vi "Create Master Instance (UDP).vi"(4 "write operation timeout":i32=1000, 6 "read operation timeout":i32=1000, 8 "error in (no error)":errorcluster, 9 "connect timeout":i32=1000, 10 "port (auto)":u16, 11 "address":string) -> (0 "error out":errorcluster, 3 "UDP master instance":refnum<class "Modbus Master.lvclass">)   [LabVIEW 2021]
doc: "Creates a serial or TCP Modbus master instance. You must manually select the polymorphic instance to use."
uses:
  Modbus Master.lvclass
  Modbus_v2/subvis/Transmission Data Unit (ADU)/IP Data Unit/IP Data Unit.lvclass
  Modbus API.lvclass
  Transmission Data Unit/Transmission Data Unit.lvclass
  Modbus_v2/subvis/Protocol/UDP/UDP Master/UDP Master.lvclass
  D:/my_projects/projects/Algorithms/Labview/21/Modbus_v21/API/Modbus API.lvclass
  D:/my_projects/projects/Algorithms/Labview/21/Modbus_v21/API/Master/Modbus Master.lvclass
  Network Protocol/Network Master/Network Master.lvclass
  D:/my_projects/projects/Algorithms/Labview/21/Modbus_v21/Network Protocol/Network Protocol.lvclass
  D:/my_projects/projects/Algorithms/Labview/21/Modbus_v21/Network Protocol/Network Master/Network Master.lvclass
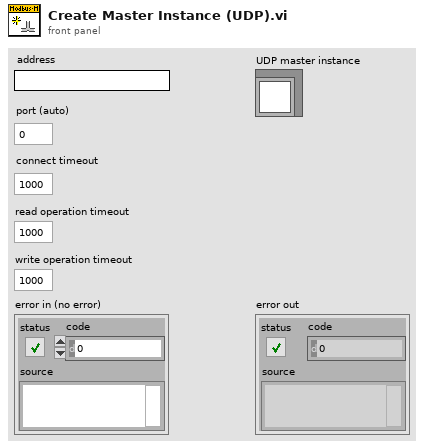
[diagram p1: front panel]
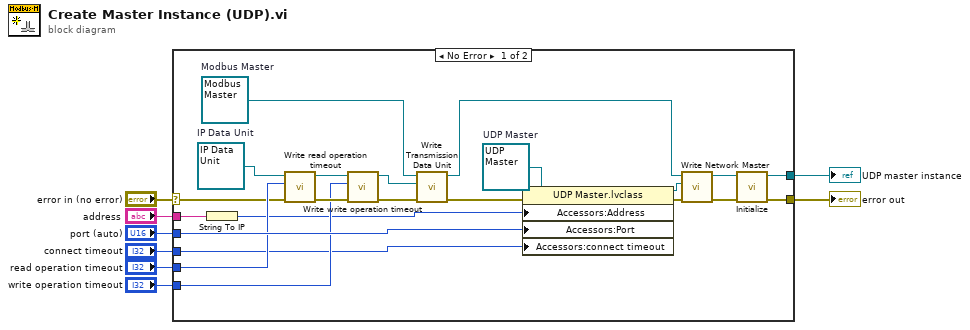
[diagram p0: block diagram]
diagram:
  n1 = case shown="No Error" "error in (no error)" {
    selector: "error in (no error)" -> [w12 w31]
    tunnel: "address" -> [w10 _]
    tunnel: "port (auto)" -> [w30 _]
    tunnel: [w29 w31] -> w1
    tunnel: [w28 _] -> w2
    tunnel: "read operation timeout" -> [w20 _]
    tunnel: "write operation timeout" -> [w19 _]
    tunnel: "connect timeout" -> [w18 _]
    frame No Error {
      w11 = refnum<class "UDP Master.lvclass"> refnum  # UDP Master
      w21 = refnum<class "IP Data Unit.lvclass"> refnum  # IP Data Unit
      w27 = refnum<class "Modbus Master.lvclass"> refnum  # Modbus Master
      n2 = String To IP(1:w10) -> (0:w9:u32)
      n3 = call "Write read operation timeout.vi"("error in (no error)"=w12, "read operation timeout"=w20, "transmission data unit in"=w21) -> ("error out"=w24:errorcluster, "transmission data unit out"=w25:refnum<class "Transmission Data Unit.lvclass">)  [unwired: 7 in]
      n4 = call "Write write operation timeout.vi"("error in (no error)"=w24, "write operation timeout"=w19, "transmission data unit in"=w25) -> ("error out"=w23:errorcluster, "transmission data unit out"=w22:refnum<class "Transmission Data Unit.lvclass">)  [unwired: 7 in]
      n5 = call "Write Transmission Data Unit.vi"("error in"=w23, "transmission data unit"=w22, "Modbus instance in"=w27) -> ("error out"=w17:errorcluster, "Modbus instance out"=w16:refnum<class "Modbus Master.lvclass">)  [unwired: 7 in]
      n6 = property class="UDP Master.lvclass"(reference=w11, error in=w17, "Accessors:Address"=w9, "Accessors:Port"=w30, "Accessors:connect timeout"=w18) -> (reference out=w26:refnum<class "UDP Master.lvclass">, error out=w15:errorcluster)
      n7 = call "Write Network Master.vi"("error in (no error)"=w15, "network master"=w26, "Modbus master in"=w16) -> ("error out"=w14:errorcluster, "Modbus master out"=w13:refnum<class "Modbus Master.lvclass">)  [unwired: 7 in]
      n8 = call-dynamic "Initialize.vi"("error in (no error)"=w14, "Modbus master in"=w13) -> ("error out"=w29:errorcluster, "Modbus master out"=w28:refnum<class "Modbus Master.lvclass">)  [unwired: 8 in]
    }
    frame Error {
    }
  }
  "error out" <- w1
  "UDP master instance" <- w2
